vi "Generate positions array.vi"(8 "Error in":errorcluster, 9 "Rows/Columns":T2={"Number of rows to generate"=6, "Number of columns to generate"=0}, 11 "Experiment Parameters":T3={"Total Number of Miniscans"=1012, "Number of Trials"=20, "Number of cycles in a trial"=344, "Number of miniscans in a frame (Y)"=44, "Number of Pixels in Miniscan (X)"=85, "Number of Frames in Each Trial"=7912, "Number of Frames in a Cycle"=23, "DwellTime (us)"=0.05, "Acquisition length (sec)"=10.0, "Variable Length"=FALSE, "Pixels in miniscan (X)"=[], "Number of lines in frame (Y)"=[]}) -> (0 "error out":errorcluster, 1 "Cancel":bool, 2 "Frames info":T1)   [LabVIEW 2020]
uses:
  Typedefs/Experiment Parameters.ctl
  <vilib>/Utility/miscctls.llb/LVPointTypeDef.ctl
  <userlib>/_OpenG.lib/array/array.llb/Sort 1D Array (I32)__ogtk.vi
  <userlib>/_OpenG.lib/array/array.llb/Remove Duplicates from 1D Array (I32)__ogtk.vi
  <userlib>/_OpenG.lib/array/array.llb/Delete Elements from 1D Array (I32)__ogtk.vi
panel:
  in  "OK":bool
  in  "Layout":i32[][](array[numeric])=[[1, 2, 2, 13], [23, 1, 9, 2], [4, 19, 21, 10], [11, 12, 20, 17], [18, 22, 7, 6], [5, 8, 15, 15]] min=1 max=100 step=1 format="Image %d"
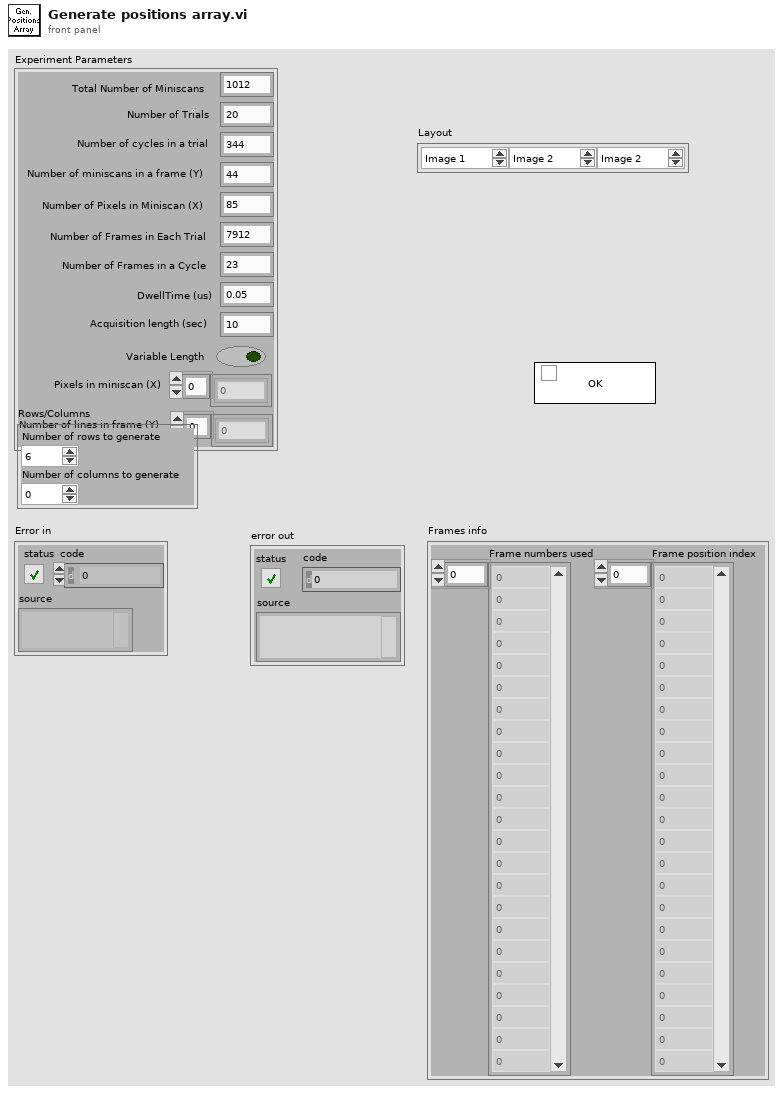
[diagram p1: front panel]
types:
  T1 = cluster{"Frame numbers used":i32[], "Frame position index":i32[]}
  T2 = cluster{"Number of rows to generate":i32, "Number of columns to generate":i32}
  T3 = typedef "Experiment Parameters.ctl" = cluster{"Total Number of Miniscans":i32, "Number of Trials":i32, "Number of cycles in a trial":i32, "Number of miniscans in a frame (Y)":i32, "Number of Pixels in Miniscan (X)":i32, "Number of Frames in Each Trial":i32, "Number of Frames in a Cycle":i32, "DwellTime (us)":dbl, "Acquisition length (sec)":dbl, "Variable Length":bool, "Pixels in miniscan (X)":dbl[], "Number of lines in frame (Y)":dbl[]}
  T4 = typedef "LVPointTypeDef.ctl" = cluster{"Horizontal":i16, "Vertical":i16}
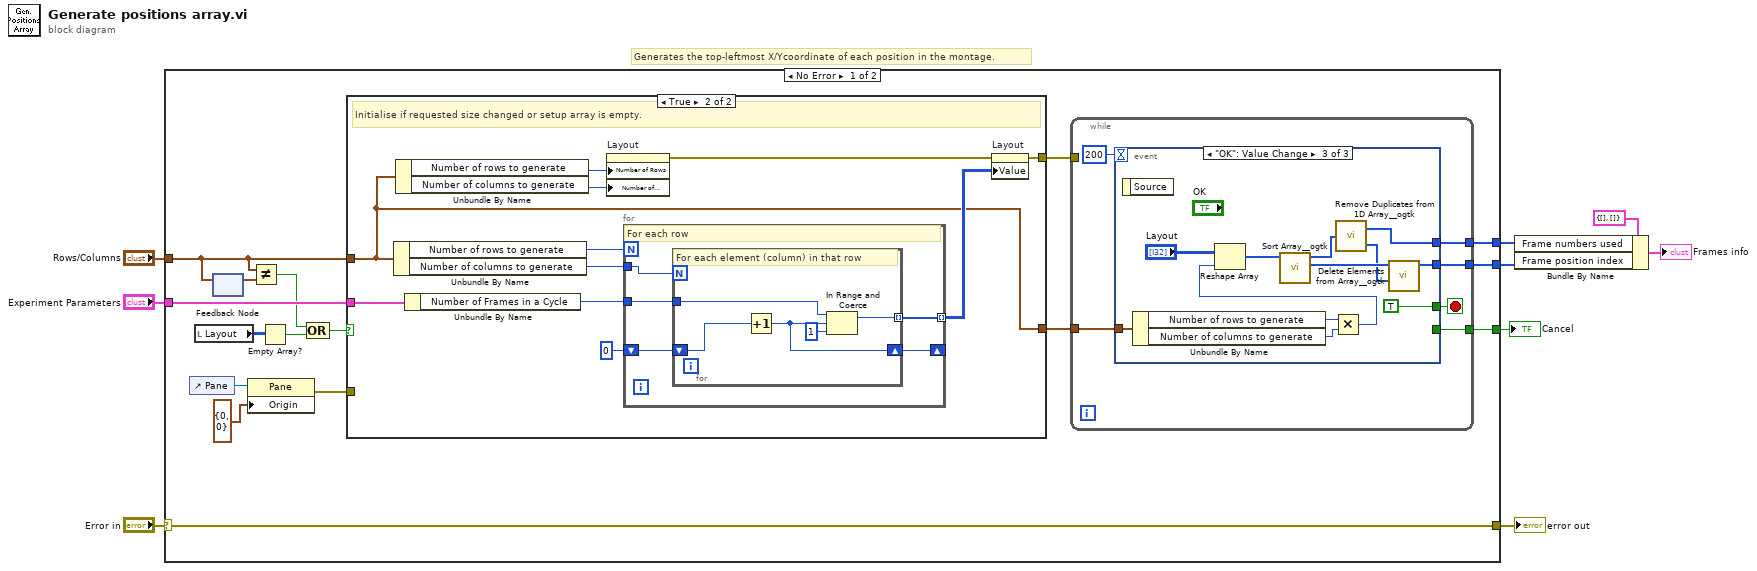
[diagram p0: block diagram]
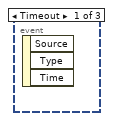
[diagram p3: hidden frame]
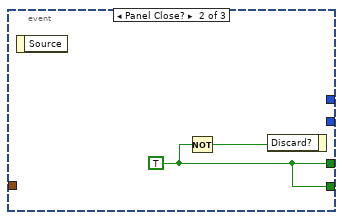
[diagram p4: hidden frame]
diagram:
  # "Generates the top-leftmost X/Ycoordinate of each position in the montage."
  n1 = case shown="No Error" "Error in" {
    selector: "Error in" -> [w25 w68]
    tunnel: "Experiment Parameters" -> [w24 _]
    tunnel: [w25 w68] -> w7
    tunnel: "Rows/Columns" -> [w17 _]
    tunnel: [w23 _] -> w3
    tunnel: [w22 _] -> w4
    tunnel: [w10 _] -> w1
    frame No Error {
      n2 = control-ref of="Pane"() -> (w13:refnum<vi>)
      n3 = local read "Layout"() -> (w20:i32[][])
      n4 = feedback-in #1(w17) -> ()
      n5 = feedback #1() -> (w18:T2)  [unwired: 1 in]
      n6 = property class="Pane"(reference=w13, "Origin"=T4 {"Horizontal"=0, "Vertical"=0}) -> (error out=w12:errorcluster)  [unwired: 1 in, 1 out]
      n7 = Not Equal?(x=w17, y=w18) -> (x != y?=w16:bool)
      n8 = Empty Array?(array=w20) -> (empty?=w19:bool)
      n9 = Compound Arithmetic op=OR(w16, w19) -> (w15:bool)
      n10 = case shown="True" w15 {
        tunnel: w24 -> [_ w37]
        tunnel: [_ w28] -> w21
        tunnel: w17 -> [w26 w27]
        tunnel: [w26 w27] -> w14
        tunnel: w12 -> [_ _]
        frame False {
          # "Do not initialise."
        }
        frame True {
          # "Initialise if requested size changed or setup array is empty."
          n11 = Unbundle By Name(w27) -> ("Number of rows to generate"=w36:i32, "Number of columns to generate"=w35:i32)
          n12 = Unbundle By Name(w27) -> ("Number of rows to generate"=w34:i32, "Number of columns to generate"=w33:i32)
          n13 = Unbundle By Name(w37) -> ("Number of Frames in a Cycle"=w31:i32)
          n14 = property on="Layout" class="Arr (strict)"("Number of Rows"=w34, "Number of Columns"=w33) -> (error out=w32:errorcluster)  [unwired: 2 in, 1 out]
          n15 = for {
            N: w36 -> [_]
            tunnel: w35 -> [w42]
            tunnel: w31 -> [w40]
            tunnel: [w41] -> w30 mode=indexing
            shift-right: [w39] -> _
            shift-left: 0 ("lower limit") -> [w38]
            # "For each row"
            n16 = for {
              N: w42 -> [_]
              tunnel: [w46] -> w41 mode=indexing
              tunnel: w40 -> [w47]
              shift-right: [w44] -> w39
              shift-left: w38 -> [w43]
              # "For each element (column) in that row"
              n17 = Increment(x=w43) -> (x+1=w44:i32)
              n18 = In Range and Coerce(upper limit=w47, x=w44, lower limit=1) -> (coerced(x)=w46:i32)  [unwired: 1 out]
            }
          }
          n19 = property on="Layout" class="Arr (strict)"(error in=w32, "Value"=w30) -> (error out=w28:errorcluster)  [unwired: 1 in, 1 out]
        }
      }
      n20 = while {
        tunnel: [w51] -> w23
        tunnel: w14 -> [w50]
        tunnel: [w49] -> w22
        tunnel: w21 -> [_]
        tunnel: [w48] -> w10
        stop <- w52 stop-if-true
        n21 = event shown="[2] \"OK\": Value Change" {
          selector: _ -> [_ _ _]
          dyn-events: _ -> [_ _ _]
          timeout: 200 -> [_ _ _]
          tunnel: [_ w54 TRUE] -> w52
          tunnel: [_ _ w58] -> w51
          tunnel: w50 -> [_ _ w64]
          tunnel: [_ _ w56] -> w49
          tunnel: [_ w54 _] -> w48
          event Timeout {
            n22 = event-data() -> ()  [unwired: 1 in, 3 out]
          }
          event Panel Close? {
            w54 = TRUE
            n23 = event-data() -> ()  [unwired: 1 in, 1 out]
            n24 = Not(x=w54) -> (.not. x?=w55:bool)
            n25 = event-data("Discard?"=w55) -> ()  [unwired: 1 in, 1 out]
          }
          event "OK": Value Change {
            n26 = event-data() -> ()  [unwired: 1 in, 1 out]
            n27 = Unbundle By Name(w64) -> ("Number of rows to generate"=w63:i32, "Number of columns to generate"=w62:i32)
            n28 = Multiply(x=w63, y=w62) -> (x*y=w66:i32)
            n29 = Reshape Array("Layout", w66) -> (w61:i32[])
            n30 = call-poly <userlib>:"Sort Array__ogtk.vi"("Array in"=w61) -> ("Sorted Pointers"=w59:i32[], "Sorted Array out"=w60:i32[])  [unwired: 9 in]
            n31 = call-poly <userlib>:"Remove Duplicates from 1D Array__ogtk.vi"("Input Array"=w60) -> ("Output Array"=w56:i32[], "indices of removed elements"=w57:i32[])
            n32 = call-poly <userlib>:"Delete Elements from Array__ogtk.vi"("indices"=w57, "array"=w59) -> ("array w/ subset deleted"=w58:i32[])  [unwired: 8 in, 1 out]
          }
        }
      }
    }
    frame Error {
    }
  }
  "error out" <- w7
  "Cancel" <- w1
  n33 = Bundle By Name(cluster=T1 {"Frame numbers used"=[], "Frame position index"=[]} ("Frames info"), "Frame numbers used"=w4, "Frame position index"=w3) -> (→"Frames info":T1)
